vi "Write Timeout.vi"(8 "error in (no error)":errorcluster, 10 "Timeout":i32=1000, 11 "RP Communicator in":refnum<class "RP Communicator VISA.lvclass">) -> (0 "error out":errorcluster, 3 "RP Communicator out":refnum<class "RP Communicator VISA.lvclass">)   [LabVIEW 2019, in "RP Communicator VISA.lvclass"]
uses:
  RP Communicator VISA.lvclass
  RP Communicator VISA.lvclass/RP Communicator VISA.ctl
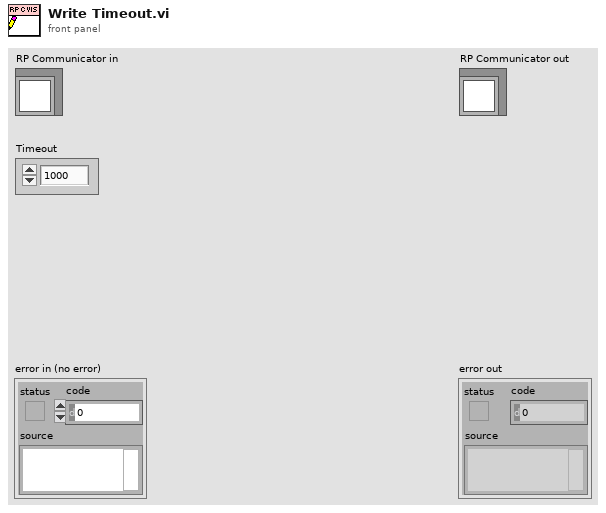
[diagram p1: front panel]
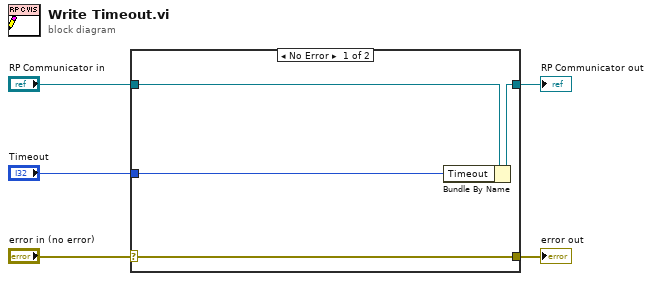
[diagram p0: block diagram]
diagram:
  n1 = case shown="No Error" "error in (no error)" {
    selector: "error in (no error)" -> [w9 w10]
    tunnel: [w9 w10] -> w4
    tunnel: [w7 w11] -> w2
    tunnel: "RP Communicator in" -> [w8 w11]
    tunnel: "Timeout" -> [w6 _]
    frame No Error {
      n2 = Bundle By Name(cluster=w8, "Timeout"=w6) -> (w7:refnum<class "RP Communicator VISA.lvclass">)
    }
    frame Error {
    }
  }
  "error out" <- w4
  "RP Communicator out" <- w2
